vi "EE_Throw EDK Error.vi"(1 "edkErrorCode":i32) -> (0 "edkErroCode":errorcluster)   [LabVIEW 2016, in "Emotiv Epoc.lvlib" / "EmotivEpocHeadsetControls.lvclass"]
doc: "Convert return codes from Emotiv API calls to LabVIEW errors."
uses:
  EmotivEpocHeadsetControls.lvclass
panel:
  # "This VI is a part of BCI Design library, http://www.ru-bci.org \nCopyright © 2020, Sotnikov Peter, All rights reserved. License: CC BY-NC 4.0"
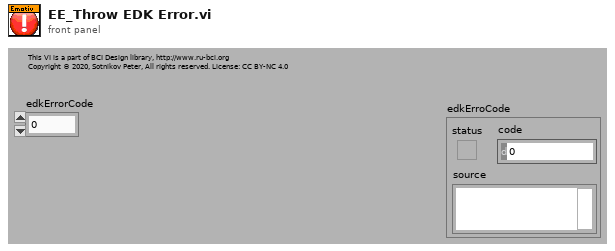
[diagram p1: front panel]
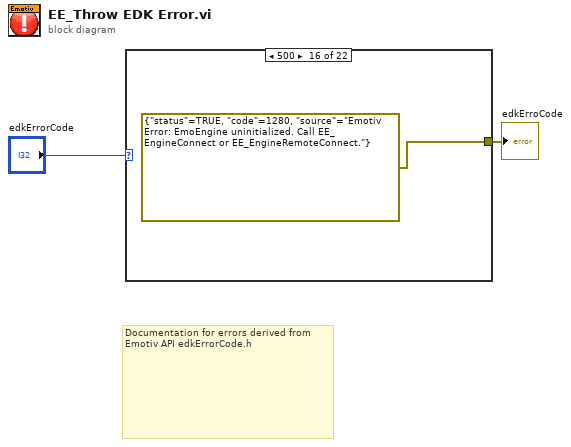
[diagram p0: block diagram]
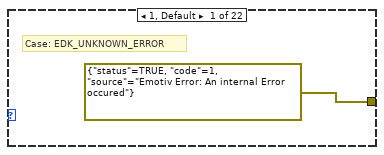
[diagram p2: hidden frame]
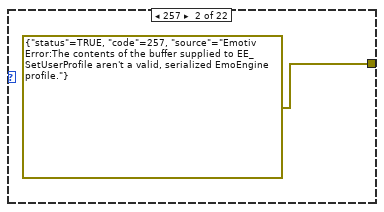
[diagram p3: hidden frame]
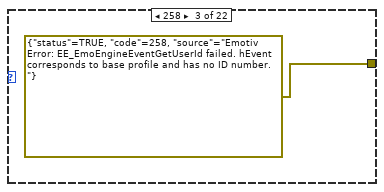
[diagram p4: hidden frame]
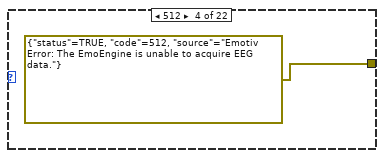
[diagram p5: hidden frame]
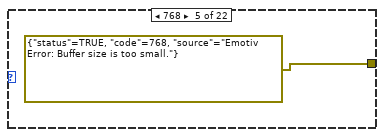
[diagram p6: hidden frame]
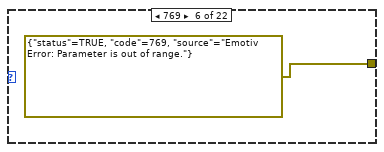
[diagram p7: hidden frame]
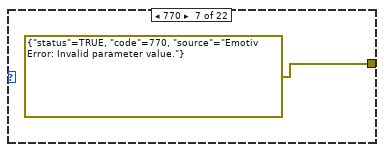
[diagram p8: hidden frame]
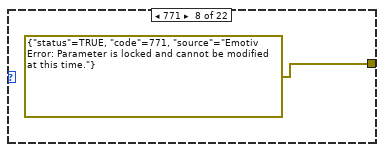
[diagram p9: hidden frame]
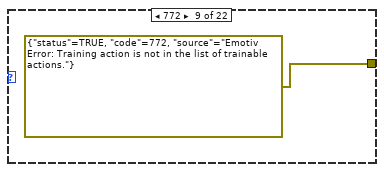
[diagram p10: hidden frame]
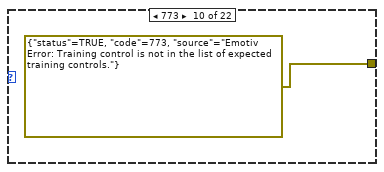
[diagram p11: hidden frame]
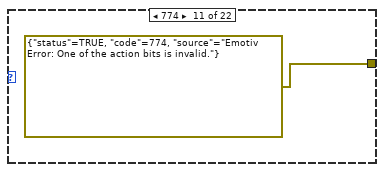
[diagram p12: hidden frame]
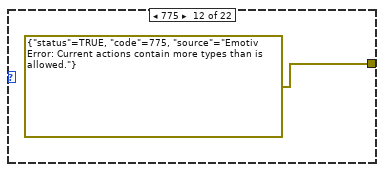
[diagram p13: hidden frame]
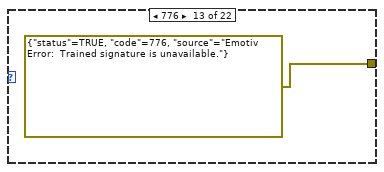
[diagram p14: hidden frame]
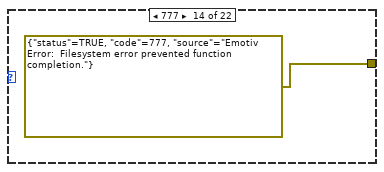
[diagram p15: hidden frame]
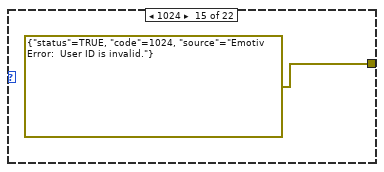
[diagram p16: hidden frame]
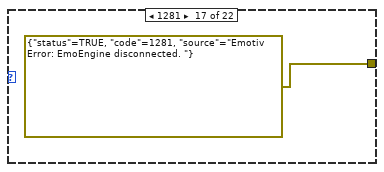
[diagram p17: hidden frame]
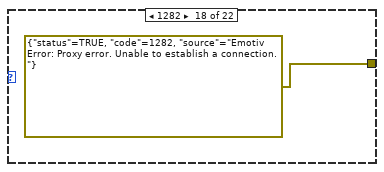
[diagram p18: hidden frame]
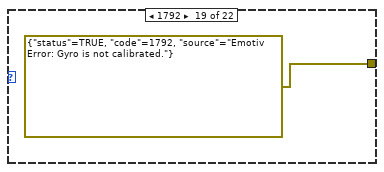
[diagram p19: hidden frame]
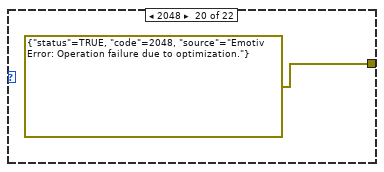
[diagram p20: hidden frame]
diagram:
  # "Documentation for errors derived from Emotiv API edkErrorCode.h"
  n1 = case shown="500" "edkErrorCode" {
    tunnel: [errorcluster {"status"=TRUE, "code"=1, "source"="Emotiv Error: An internal Error occured"} ("error out") errorcluster {"status"=TRUE, "code"=257, "source"="Emotiv Error:The contents of the buffer supplied to EE_SetUserProfile aren't a valid, serialized EmoEngine profile."} ("error out") errorcluster {"status"=TRUE, "code"=258, "source"="Emotiv Error: EE_EmoEngineEventGetUserId failed. hEvent corresponds to base profile and has no ID number."} ("error out") errorcluster {"status"=TRUE, "code"=512, "source"="Emotiv Error: The EmoEngine is unable to acquire EEG data."} ("error out") errorcluster {"status"=TRUE, "code"=768, "source"="Emotiv Error: Buffer size is too small."} ("error out") errorcluster {"status"=TRUE, "code"=769, "source"="Emotiv Error: Parameter is out of range."} ("error out") errorcluster {"status"=TRUE, "code"=770, "source"="Emotiv Error: Invalid parameter value."} ("error out") errorcluster {"status"=TRUE, "code"=771, "source"="Emotiv Error: Parameter is locked and cannot be modified at this time."} ("error out") errorcluster {"status"=TRUE, "code"=772, "source"="Emotiv Error: Training action is not in the list of trainable actions."} ("error out") errorcluster {"status"=TRUE, "code"=773, "source"="Emotiv Error: Training control is not in the list of expected training controls."} ("error out") errorcluster {"status"=TRUE, "code"=774, "source"="Emotiv Error: One of the action bits is invalid."} ("error out") errorcluster {"status"=TRUE, "code"=775, "source"="Emotiv Error: Current actions contain more types than is allowed."} ("error out") errorcluster {"status"=TRUE, "code"=776, "source"="Emotiv Error:  Trained signature is unavailable."} ("error out") errorcluster {"status"=TRUE, "code"=777, "source"="Emotiv Error:  Filesystem error prevented function completion."} ("error out") errorcluster {"status"=TRUE, "code"=1024, "source"="Emotiv Error:  User ID is invalid."} ("error out") errorcluster {"status"=TRUE, "code"=1280, "source"="Emotiv Error: EmoEngine uninitialized. Call EE_EngineConnect or EE_EngineRemoteConnect."} ("error out") errorcluster {"status"=TRUE, "code"=1281, "source"="Emotiv Error: EmoEngine disconnected. "} ("error out") errorcluster {"status"=TRUE, "code"=1282, "source"="Emotiv Error: Proxy error. Unable to establish a connection."} ("error out") errorcluster {"status"=TRUE, "code"=1792, "source"="Emotiv Error: Gyro is not calibrated."} ("error out") errorcluster {"status"=TRUE, "code"=2048, "source"="Emotiv Error: Operation failure due to optimization."} ("error out") errorcluster {"status"=TRUE, "code"=2304, "source"="Emotiv Error: Reserved return value."} ("error out") errorcluster {"status"=FALSE, "code"=0, "source"=""} ("error IO")] -> w1
    frame 1, Default {
      # "Case: EDK_UNKNOWN_ERROR"
    }
    frame 257 {
    }
    frame 258 {
    }
    frame 512 {
    }
    frame 768 {
    }
    frame 769 {
    }
    frame 770 {
    }
    frame 771 {
    }
    frame 772 {
    }
    frame 773 {
    }
    frame 774 {
    }
    frame 775 {
    }
    frame 776 {
    }
    frame 777 {
    }
    frame 1024 {
    }
    frame 1280 {
    }
    frame 1281 {
    }
    frame 1282 {
    }
    frame 1792 {
    }
    frame 2048 {
    }
    frame 2304 {
    }
    frame 0, 1536 {
      # "Case: EDK_NO_EVENT"
      # "Case: EDK_OK"
    }
  }
  "edkErroCode" <- w1
